vi "appendTable--string.vi"(8 "error in (no error)":errorcluster, 9 "Font":refnum<class "Style.lvclass">, 10 "Table":string[][](array[string]), 11 "MS-Word in":refnum<class "MS-Word.lvclass">) -> (0 "error out":errorcluster, 3 "MS-Word out":refnum<class "MS-Word.lvclass">)   [LabVIEW 2017, in "LabVIEW NPOI.lvlib" / "MS-Word.lvclass"]
doc: "Protected dynamic dispatch method to append the wire <b>Table</b> as 2D array of strings to the <b>Document</b> as a table."
uses:
  MS-Word.lvclass
  Styles/Style/Style.lvclass
  MS-Word.lvclass/MS-Word.ctl
  xwpfDocument/xwpfDocument.lvclass
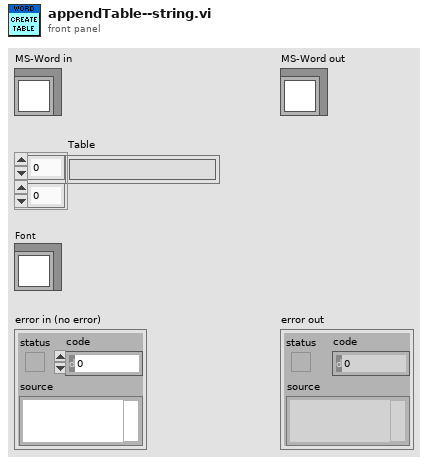
[diagram p1: front panel]
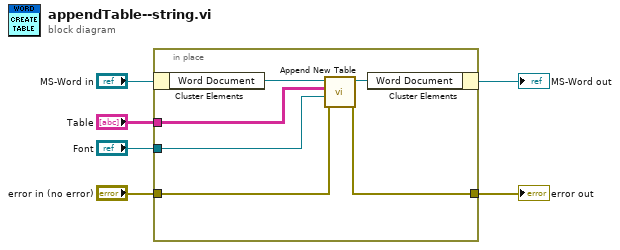
[diagram p0: block diagram]
diagram:
  n1 = in-place {
    in-place-border: "Table" -> [w9]
    in-place-border: "error in (no error)" -> [w8]
    in-place-border: [w7] -> w3
    in-place-border: "Font" -> [w10]
    n2 = in-place-cluster #1("MS-Word in") -> ("Word Document"=w12:refnum<class "xwpfDocument.lvclass">)
    n3 = call "Append New Table.vi"("error in (no error)"=w8, "Cell.Style"=w10, "Table.Data"=w9, "xwpfDocument in"=w12) -> ("error out"=w7:errorcluster, "xwpfDocument out"=w11:refnum<class "xwpfDocument.lvclass">)  [unwired: 6 in]
    n4 = in-place-cluster #1("Word Document"=w11) -> (→"MS-Word out":refnum<class "MS-Word.lvclass">)
  }
  "error out" <- w3
